vi "calc_Actuators_setSetPoint.vi"(8 "Throttle Deadband (0.1)":dbl, 9 "Fixed Intake Angle":dbl, 10 "Joystick Axis Value":dbl) -> (3 "Angle Setpoint":dbl)   [LabVIEW 2017]
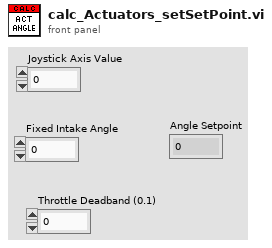
[diagram p1: front panel]
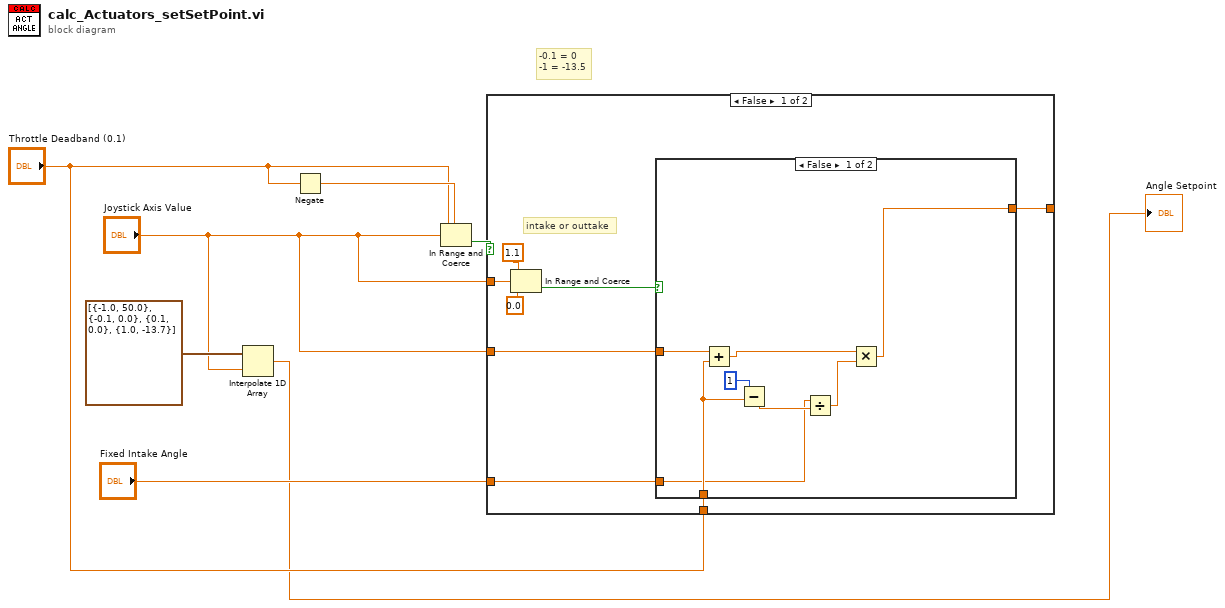
[diagram p0: block diagram]
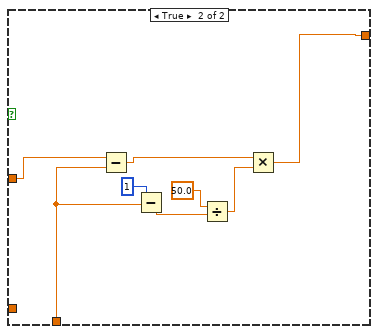
[diagram p2: hidden frame]
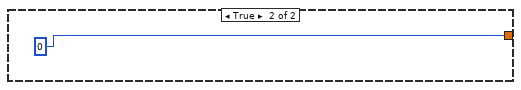
[diagram p3: hidden frame]
diagram:
  # "-0.1 = 0 \n-1 = -13.5"
  n1 = Interpolate 1D Array(1:"Joystick Axis Value", 2:cluster{dbl, dbl}[] [{-1.0, 50.0}, {-0.1, 0.0}, {0.1, 0.0}, {1.0, -13.7}]) -> (0:→"Angle Setpoint":dbl)
  n2 = Negate(x="Throttle Deadband (0.1)") -> (-x=w6:dbl)
  n3 = In Range and Coerce(upper limit="Throttle Deadband (0.1)", x="Joystick Axis Value", lower limit=w6) -> (In Range?=w7:bool)  [unwired: 1 out]
  n4 = case shown="False" w7 {
    tunnel: "Joystick Axis Value" -> [w15 _]
    tunnel: "Joystick Axis Value" -> [w11 _]
    tunnel: "Throttle Deadband (0.1)" -> [w10 _]
    tunnel: [w8 0] -> _
    tunnel: "Fixed Intake Angle" -> [w9 _]
    frame False {
      # "intake or outtake"
      n5 = In Range and Coerce(upper limit=1.1, x=w15, lower limit=0.0) -> (In Range?=w12:bool)  [unwired: 1 out]
      n6 = case shown="False" w12 {
        tunnel: w11 -> [w23 w27]
        tunnel: w10 -> [w21 w26]
        tunnel: [w17 w24] -> w8
        tunnel: w9 -> [w16 _]
        frame False {
          n7 = Add(x=w23, y=w21) -> (x+y=w19:dbl)
          n8 = Subtract(x=1, y=w21) -> (x-y=w20:dbl)
          n9 = Divide(x=w16, y=w20) -> (x/y=w18:dbl)
          n10 = Multiply(x=w19, y=w18) -> (x*y=w17:dbl)
        }
        frame True {
          n11 = Subtract(x=w27, y=w26) -> (x-y=w30:dbl)
          n12 = Subtract(x=1, y=w26) -> (x-y=w29:dbl)
          n13 = Divide(x=50.0, y=w29) -> (x/y=w31:dbl)
          n14 = Multiply(x=w30, y=w31) -> (x*y=w24:dbl)
        }
      }
    }
    frame True {
    }
  }
